vi "tb_U16 Shifter by 2.vi"() -> ()   [LabVIEW 2011]
panel:
  out "interleaved array":dbl[](array[numeric])
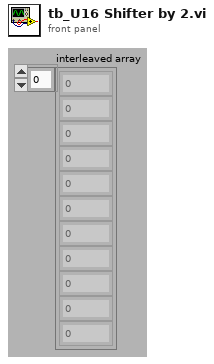
[diagram p1: front panel]
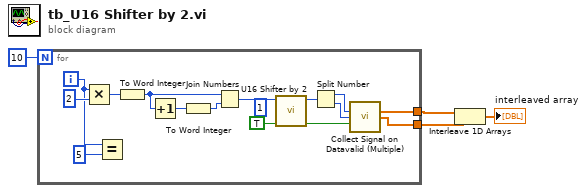
[diagram p0: block diagram]
diagram:
  n1 = for {
    N: 10 -> [_]
    tunnel: [w9] -> w3
    tunnel: [w8] -> w2
    i -> [w7]
    (unwired) u8 1 ("Shift")
    n2 = Multiply(x=w7, y=2) -> (x*y=w17:i32)
    n3 = Equal?(x=w7, y=5) -> ()  [unwired: 1 out]
    n4 = To Word Integer(number=w17) -> (16bit integer=w5:i16)
    n5 = Increment(x=w5) -> (x+1=w18:i16)
    n6 = To Word Integer(number=w18) -> (16bit integer=w16:i16)
    n7 = Join Numbers(hi=w5, lo=w16) -> ((hi.lo)=w15:u32)
    n8 = call <userlib>:"U16 Shifter by 2.vi"("Input Valid"=TRUE, "Current Data"=w15) -> ("Output Data Valid"=w10:bool, "Shifted Data"=w13:u32)  [unwired: 8 in]
    n9 = Split Number(x=w13) -> (hi(x)=w12:u16, lo(x)=w11:u16)
    n10 = call <userlib>:"Collect Signal on Datavalid (Multiple).vi"("Input 1"=w12, "Input 2"=w11, "Data Valid"=w10) -> ("Output 1"=w9:dbl[], "Output 2"=w8:dbl[])  [unwired: 11 in]
  }
  n11 = Interleave 1D Arrays(w3, w2) -> (→"interleaved array":dbl[])
